vi "Histogram Mean & Standard Deviation.vi"(8 "Error In":errorcluster, 10 "Histogram":dbl[](array[numeric]), 11 "Values":dbl[](array[numeric])) -> (0 "Error Out":errorcluster, 1 "Histogram Sum":dbl, 2 "Standard Deviation":dbl, 3 "Mean":dbl)   [LabVIEW 2021, in "Histogram Window.lvlib"]
uses:
  <vilib>/Utility/error.llb/Error Cluster From Error Code.vi
  <vilib>/ErrorRing/Error Ring.xnode
  Histogram Window.lvlib
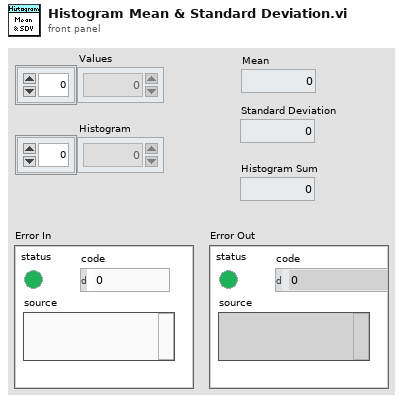
[diagram p1: front panel]
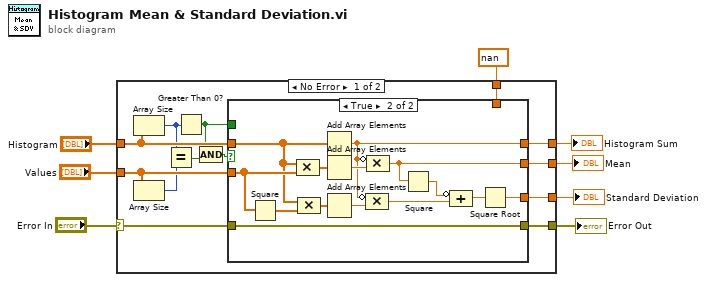
[diagram p0: block diagram]
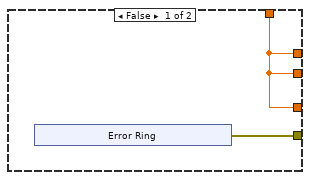
[diagram p2: hidden frame]
diagram:
  n1 = case shown="No Error" "Error In" {
    selector: "Error In" -> [w9 w42]
    tunnel: [w21 w43] -> w8
    tunnel: [w20 w43] -> w7
    tunnel: [w19 w43] -> w6
    tunnel: "Values" -> [w18 _]
    tunnel: "Histogram" -> [w17 _]
    tunnel: nan ("Numeric Control") -> [w12 w43]
    tunnel: [w10 w42] -> w1
    frame No Error {
      n2 = Array Size(array=w17) -> (size(s)=w14:i32)
      n3 = Array Size(array=w18) -> (size(s)=w16:i32)
      n4 = Equal?(x=w14, y=w16) -> (x = y?=w15:bool)
      n5 = Greater Than 0?(x=w14) -> (x > 0?=w11:bool)
      n6 = Compound Arithmetic op=AND(w11, w15) -> (w13:bool)
      n7 = case shown="True" w13 {
        tunnel: [w23 w37] -> w21
        tunnel: [w23 w36] -> w20
        tunnel: [w23 w32] -> w19
        tunnel: w18 -> [_ w31]
        tunnel: w17 -> [_ w30]
        tunnel: w12 -> [w23 _]
        tunnel: w11 -> [_ _]
        tunnel: [w22 w28] -> w10
        tunnel: w9 -> [_ w28]
        frame False {
          n8 = xnode "Error Ring"() -> ("error out"=w22:errorcluster)
        }
        frame True {
          n9 = Square(x=w31) -> (x^2=w39:dbl[])
          n10 = Compound Arithmetic op=MULTIPLY(w30, w31) -> (w41:dbl[])
          n11 = Compound Arithmetic op=MULTIPLY(w30, w39) -> (w38:dbl[])
          n12 = Add Array Elements(numeric array=w30) -> (sum=w37:dbl)
          n13 = Add Array Elements(numeric array=w41) -> (sum=w40:dbl)
          n14 = Add Array Elements(numeric array=w38) -> (sum=w29:dbl)
          n15 = Compound Arithmetic op=MULTIPLY(invert w37, w29) -> (w35:dbl)
          n16 = Compound Arithmetic op=MULTIPLY(invert w37, w40) -> (w36:dbl)
          n17 = Square(x=w36) -> (x^2=w34:dbl)
          n18 = Compound Arithmetic op=ADD(invert w34, w35) -> (w33:dbl)
          n19 = Square Root(x=w33) -> (sqrt(x)=w32:dbl)
        }
      }
    }
    frame Error {
    }
  }
  "Mean" <- w7
  "Standard Deviation" <- w6
  "Histogram Sum" <- w8
  "Error Out" <- w1
